vi "array_add_literal.vi"(10 "bank":dbl[](array[numeric])) -> (2 "result":dbl[](array[numeric]))   [LabVIEW 2020]
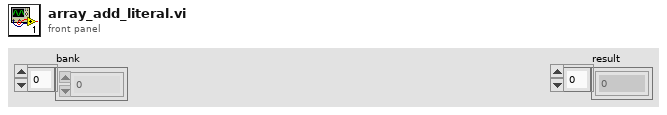
[diagram p1: front panel]
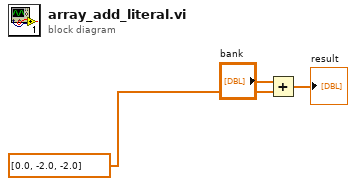
[diagram p0: block diagram]
diagram:
  n1 = Add(x="bank", y=dbl[] [0.0, -2.0, -2.0]) -> (x+y=→"result":dbl[])
